vi "Error - Fire Error.vi"(8 "error in (no error)":errorcluster, 10 "Error Type":T1, 11 "View Model":T2) -> (0 "error out":errorcluster, 3 "View Model":T2)   [LabVIEW 2017]
doc: "Generates error with parameters"
uses:
  View Model/Controls/View Model.ctl
  Configuration/Controls/Config Model.ctl
  Configuration/Controls/Config Data.ctl
  Controls/Error Model.ctl
  Controls/Error Data.ctl
  Controls/Error Type.ctl
  View Model/Controls/Shared Model.ctl
  Elevator Controller/Controls/Elevator Model.ctl
  Elevator Controller/Controls/Elevator Location.ctl
  Elevator Controller/Controls/Elevator CMD Data.ctl
  Elevator Controller/Controls/Elevator Commands.ctl
  Elevator Controller/Controls/Elevator Overhead.ctl
  Elevator Controller/Controls/Elevator States.ctl
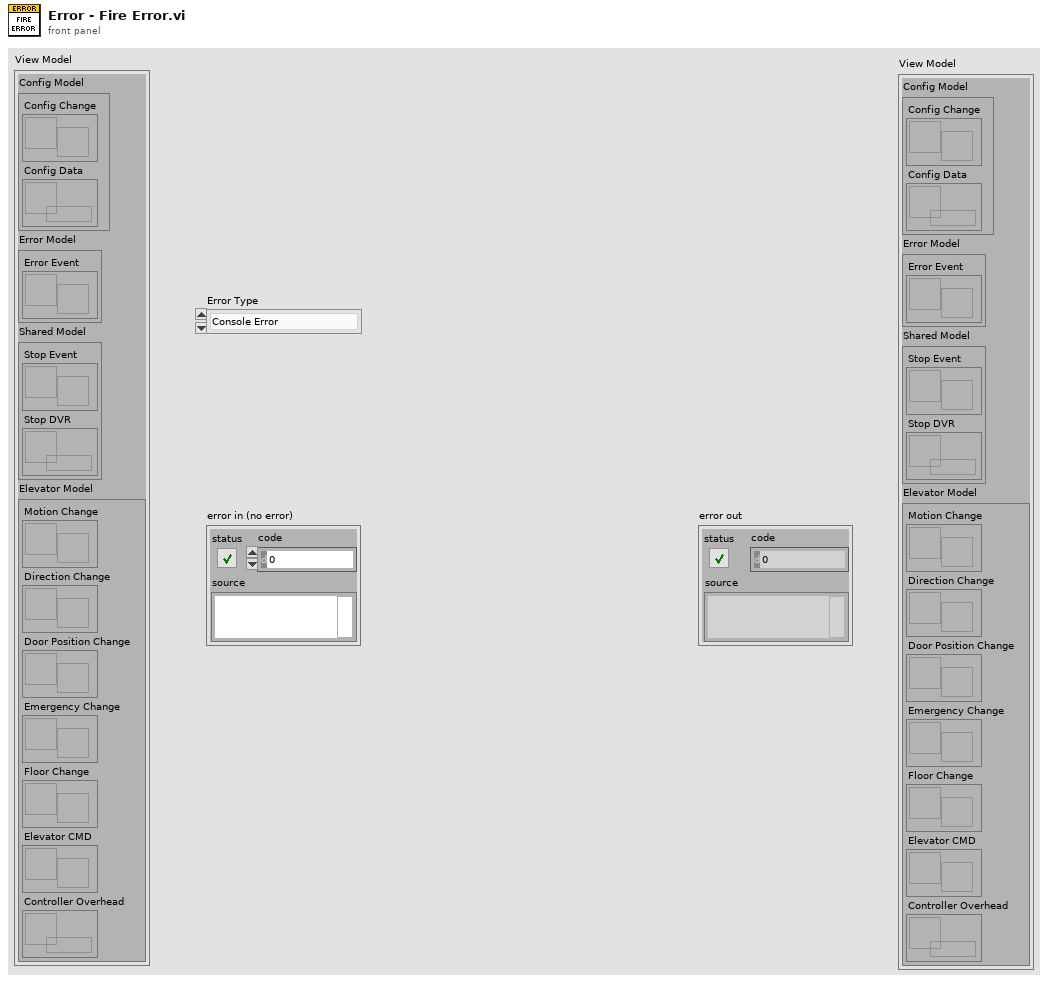
[diagram p1: front panel]
types:
  T1 = typedef "Error Type.ctl" = enum16{"Console Error", "Process Step Error", "Sensor Interface IO Error"}
  T2 = typedef "View Model.ctl" = cluster{"Config Model":T3, "Error Model":T4, "Shared Model":T5, "Elevator Model":T6}
  T3 = typedef "Config Model.ctl" = cluster{"Config Change":refnum<user-event>, "Config Data":refnum<data-value>}
  T4 = typedef "Error Model.ctl" = cluster{"Error Event":refnum<user-event>}
  T5 = typedef "Shared Model.ctl" = cluster{"Stop Event":refnum<user-event>, "Stop DVR":refnum<data-value>}
  T6 = typedef "Elevator Model.ctl" = cluster{"Motion Change":refnum<user-event>, "Direction Change":refnum<user-event>, "Door Position Change":refnum<user-event>, "Emergency Change":refnum<user-event>, "Floor Change":refnum<user-event>, "Elevator CMD":refnum<user-event>, "Controller Overhead":refnum<data-value>}
  T7 = typedef "Error Data.ctl" = cluster{"Error Type":T1, "Variant":variant}
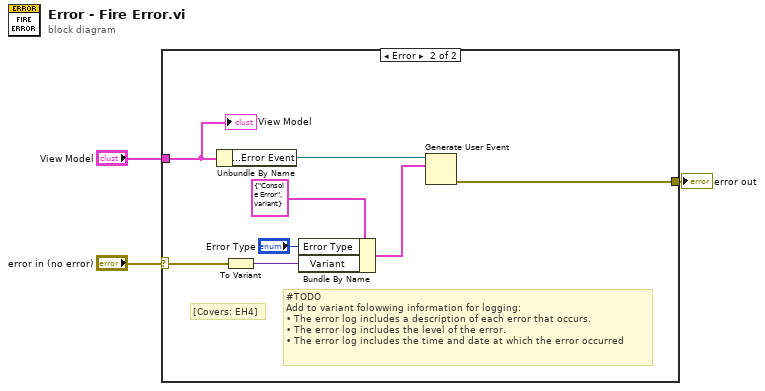
[diagram p0: block diagram]
diagram:
  n1 = case shown="Error" "error in (no error)" {
    selector: "error in (no error)" -> [w4 w5]
    tunnel: "View Model" -> [_ w7]
    tunnel: [w4 w6] -> w1
    frame No Error {
    }
    frame Error {
      # "[Covers: EH4]"
      # "#TODO\nAdd to variant folowwing information for logging:\n• The error log includes a description of each error that occurs.\n• The error log includes the level of the error.\n• The error log includes the time and date at which the error occurred"
      n2 = Unbundle By Name(w7) -> ("Error Model.Error Event"=w12:refnum<user-event>)
      n3 = To Variant(anything=w5) -> (Variant=w10:variant)
      n4 = Bundle By Name(cluster=T7 {"Error Type"=enum."Console Error", "Variant"=variant} ("Error Data"), "Error Type"="Error Type", "Variant"=w10) -> (w8:T7)
      n5 = Generate User Event(user event=w12, event data cluster=w8) -> (error out=w6:errorcluster)  [unwired: 2 in, 1 out]
      "View Model" <- w7
    }
  }
  "error out" <- w1
